vi "triggered scope simple.vi"() -> ()   [LabVIEW 2014]
uses:
  <vilib>/Utility/file.llb/Write To Spreadsheet File (DBL).vi
  <instrlib>/Tektronix TDS 200 1000 2000 Series/Public/Configure/Configure Trigger (Edge).vi
  <instrlib>/Tektronix TDS 200 1000 2000 Series/Public/Data/Read (Multiple Waveforms).vi
  <vilib>/Waveform/WDTOps.llb/WDT Waveform to XY Pairs DBL.vi
  <vilib>/Utility/file.llb/Write To Spreadsheet File (string).vi
  <instrlib>/Tektronix TDS 200 1000 2000 Series/Tektronix TDS 200 1000 2000 Series.lvlib
panel:
  in  "Pulse generator":T1={"Delay"={"A offset (s)"=0.0, "A reference"=enum."T0", "B reference"=enum."T0", "B offset (s)"=0.0, "C reference"=enum."T0", "C offset (s)"=0.0, "D reference"=enum."T0", "D offset (s)"=0.0}, "Trigger"={"Trigger"=enum."internal", "Burst count"=0, "Burst period"=0, "Input impedance"=FALSE, "Trigger slope"=FALSE, "Internal trigger rate"=0.001}, "Output"={"Mode"=enum."TTL", "Load"=FALSE, "Invert?"=FALSE, "Amplitude (V)"=2.0, "Offset (V)"=0.0, "Set output"=3}, "output cluster"={"mode"=0, "load"=FALSE, "inversion"=FALSE, "amplitude"=0.0, "offset"=0.0}} {"Output"."Set output" items=["T0", "A", "B", "AB", "C", "D", "CD"]; "Trigger"."Internal trigger rate" format="%#.9f"; "Trigger"."Burst period" max=1000 step=1; "Trigger"."Burst count" max=1000 step=1; "Delay"."D offset (s)" min=0.0 max=1.0; "Delay"."C offset (s)" min=0.0 max=1.0; "Delay"."B offset (s)" min=0.0 max=1.0; "Delay"."A offset (s)" min=0.0 max=1.0}
  out "File path":path
  in  "Tektronix scope":T2={"Trigger"={" Source"=4, "Level (V)"=0.5, "Trigger Mode"=1, "Trigger Coupling"=1, "Trigger on?"=TRUE}, "Channel 1"={"V/div"=2.0, " offset (V)"=0.0}, "Channel 2"={"V/div"=2.0, " offset (V)"=0.0}, "Time base"={"s/div"=0.003, " offset (s)"=0.0}} {"Time base"."offset (s)" min=-1.0 max=1.0; "Time base"."s/div" min=2.5e-09 max=50.0; "Channel 2"."offset (V)" min=-20.0 max=20.0; "Channel 2"."V/div" min=0.02 max=50.0; "Channel 1"."offset (V)" min=-20.0 max=20.0; "Channel 1"."V/div" min=0.02 max=50.0; "Trigger"."Trigger Coupling" items=["AC", "DC", "HF Reject", "LF Reject", "Noise Reject"]; "Trigger"."Trigger Mode" items=["Auto", "Normal"]; "Trigger"."Level (V)" min=0.0 max=4.0; "Trigger"."Source" items=["Channel 1", "Channel 2", "Channel 3", "Channel 4", "External Input", "Attenuated External Input"]}
  out "Waveform Graph":waveform(dbl)[](graph)
  in  "Stop Button":bool
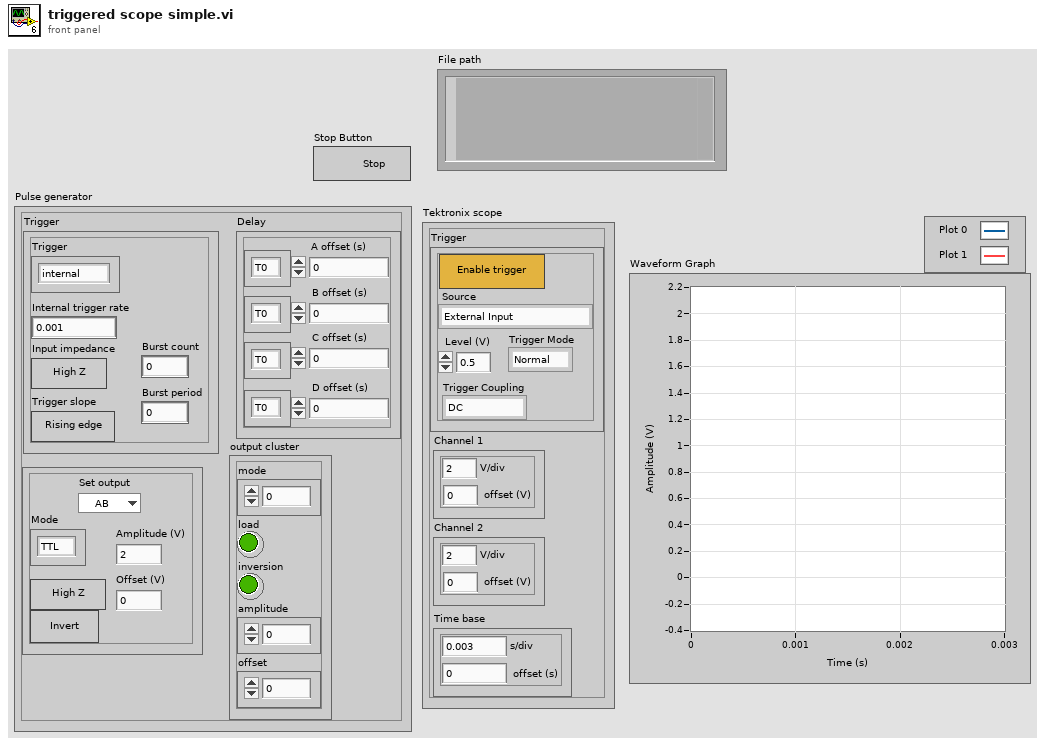
[diagram p1: front panel]
types:
  T1 = cluster{"Delay":cluster{"A offset (s)":dbl, "A reference":enum16{"T0", "B", "C", "D"}, "B reference":enum16{"T0", "A", "C", "D"}, "B offset (s)":dbl, "C reference":enum16{"T0", "A", "B", "D"}, "C offset (s)":dbl, "D reference":enum16{"T0", "A", "B", "C"}, "D offset (s)":dbl}, "Trigger":cluster{"Trigger":enum16{"internal", "external", "single shot", "burst", "line"}, "Burst count":u32, "Burst period":u32, "Input impedance":bool, "Trigger slope":bool, "Internal trigger rate":dbl}, "Output":cluster{"Mode":enum16{"TTL", "NIM", "ECL", "VAR"}, "Load":bool, "Invert?":bool, "Amplitude (V)":dbl, "Offset (V)":dbl, "Set output":u16}, "output cluster":cluster{"mode":u8, "load":bool, "inversion":bool, "amplitude":dbl, "offset":dbl}}
  T2 = cluster{"Trigger":cluster{" Source":i32, "Level (V)":dbl, "Trigger Mode":i32, "Trigger Coupling":i32, "Trigger on?":bool}, "Channel 1":cluster{"V/div":dbl, " offset (V)":dbl}, "Channel 2":cluster{"V/div":dbl, " offset (V)":dbl}, "Time base":cluster{"s/div":dbl, " offset (s)":dbl}}
  T3 = cluster{"Trigger":enum16{"internal", "external", "single shot", "burst", "line"}, "Burst count":u32, "Burst period":u32, "Input impedance":bool, "Trigger slope":bool, "Internal trigger rate":dbl}
  T4 = cluster{"A offset (s)":dbl, "A reference":enum16{"T0", "B", "C", "D"}, "B reference":enum16{"T0", "A", "C", "D"}, "B offset (s)":dbl, "C reference":enum16{"T0", "A", "B", "D"}, "C offset (s)":dbl, "D reference":enum16{"T0", "A", "B", "C"}, "D offset (s)":dbl}
  T5 = cluster{"Mode":enum16{"TTL", "NIM", "ECL", "VAR"}, "Load":bool, "Invert?":bool, "Amplitude (V)":dbl, "Offset (V)":dbl, "Set output":u16}
  T6 = enum16{"internal", "external", "single shot", "burst", "line"}
  T7 = cluster{" Source":i32, "Level (V)":dbl, "Trigger Mode":i32, "Trigger Coupling":i32, "Trigger on?":bool}
  T8 = cluster{"mode":u8, "load":bool, "inversion":bool, "amplitude":dbl, "offset":dbl}
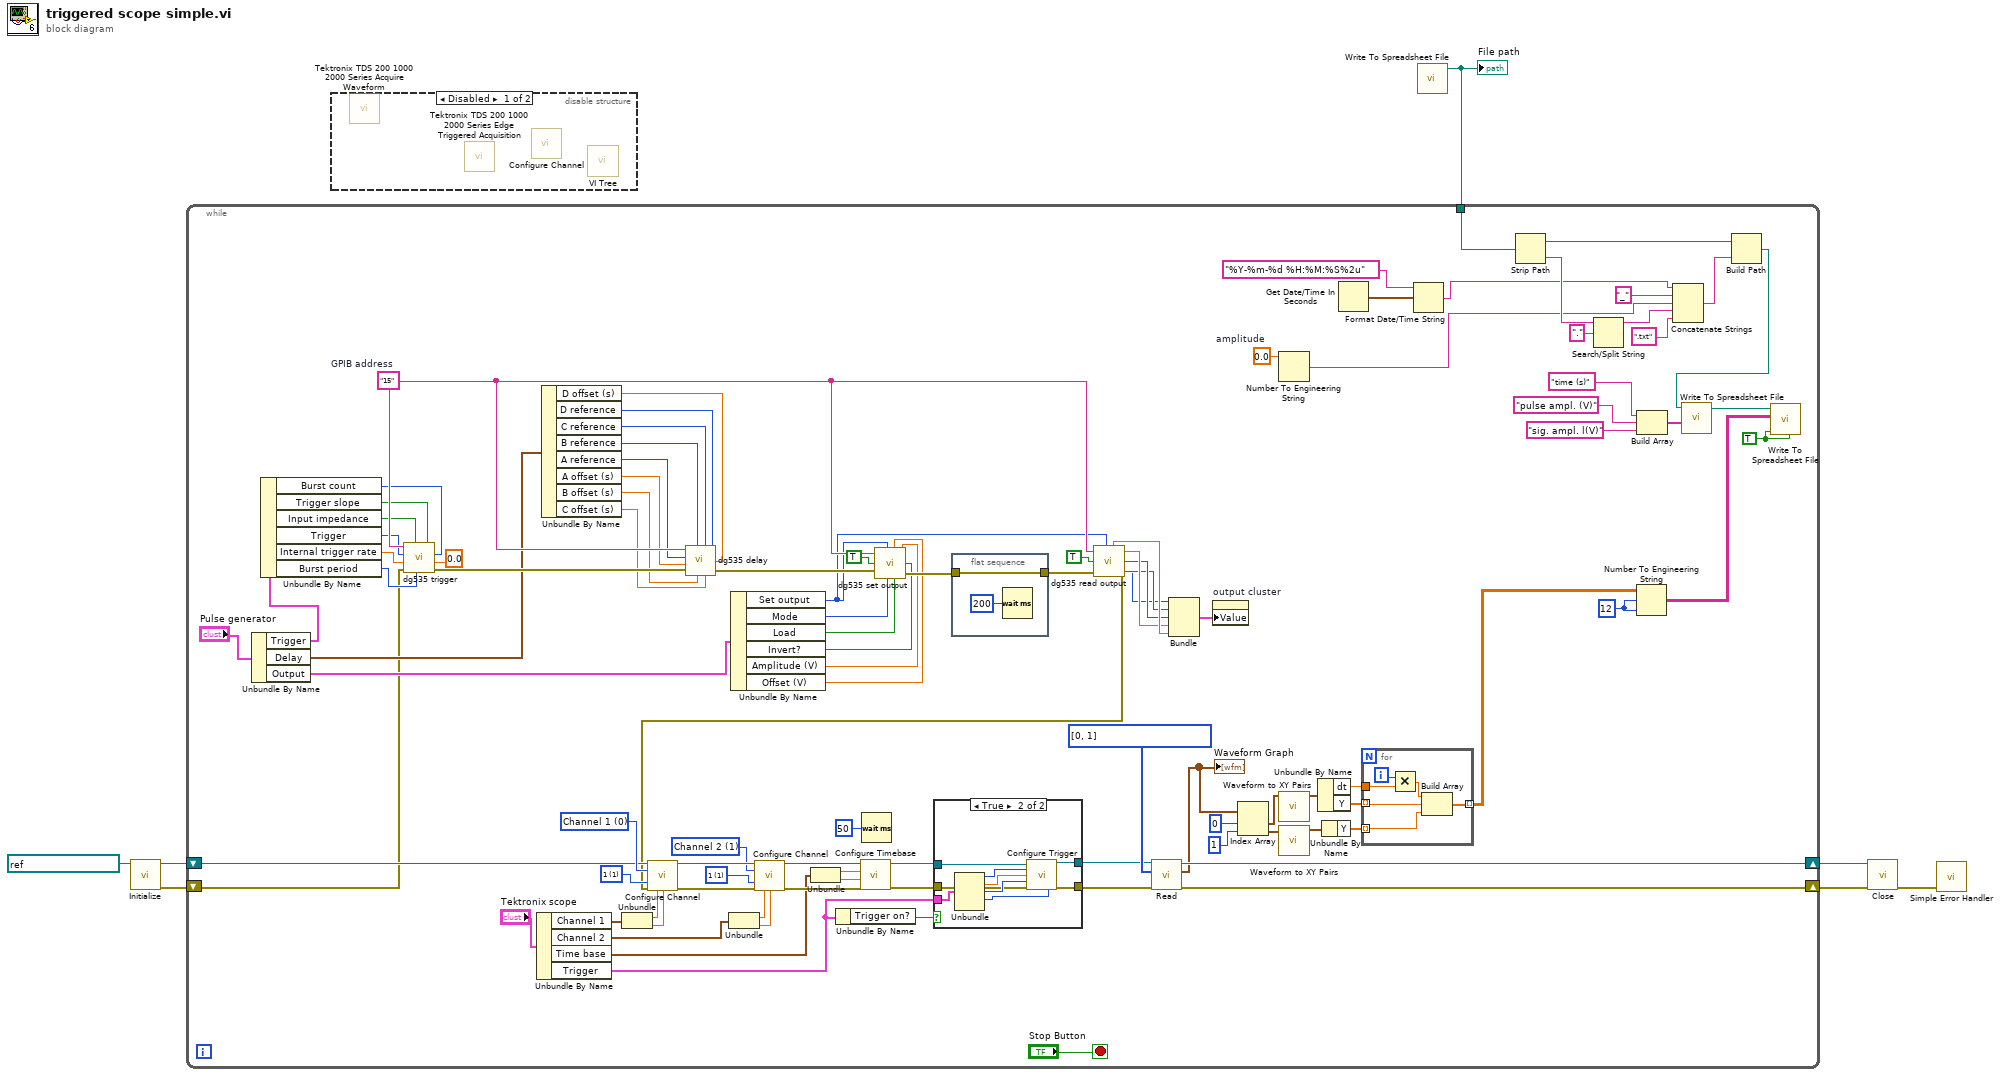
[diagram p0: block diagram]
diagram:
  n1 = call <instrlib>:"Initialize.vi"("VISA resource name"=refnum<visa-resource-name> "GPIB2::20::INSTR") -> ("error out"=w5:errorcluster, "VISA resource name out"=w6:refnum<visa-resource-name>)  [unwired: 9 in]
  n2 = disable-structure shown="Disabled" {
    frame Disabled {
      n3 = call "Tektronix TDS 200 1000 2000 Series Acquire Waveform.vi"() -> ()  [unwired: 1 in]
      n4 = call "Tektronix TDS 200 1000 2000 Series Edge Triggered Acquisition.vi"() -> ()  [unwired: 1 in]
      n5 = call <instrlib>:"Configure Channel.vi"() -> ()  [unwired: 14 in, 2 out]
      n6 = call "VI Tree.vi"() -> ()  [unwired: 12 in]
    }
    frame Enabled {
    }
  }
  n7 = call-poly <vilib>:"Write To Spreadsheet File.vi"() -> ("new file path (Not A Path if cancelled)"=w1:path)  [unwired: 8 in]
  "File path" <- w1
  n8 = while {
    shift-right: [w110] -> w7
    shift-left: w6 -> [w95]
    shift-right: [w109] -> w4
    shift-left: w5 -> [w9]
    tunnel: w1 -> [w57]
    stop <- "Stop Button" stop-if-true
    w36 = "15"  # GPIB address
    w48 = i16 12 ("width (-)")
    w52 = 0.0  # amplitude
    w58 = TRUE ("append to file? (new file:F)")
    w85 = 1 items=["1"=1, "10"=10, "20"=20, "50"=50, "100"=100, "500"=500, "1000"=1000] ("Probe Attenuation (10: 10X)")
    w87 = 1 items=["1"=1, "10"=10, "20"=20, "50"=50, "100"=100, "500"=500, "1000"=1000] ("Probe Attenuation (10: 10X)")
    w86 = u16 1 items=["Channel 1", "Channel 2", "Channel 3", "Channel 4", "Math", "Reference A", "Reference B", "Reference C", "Reference D", "FFT"] ("Source (0: Channel 1)")
    w100 = u16 0 items=["Channel 1", "Channel 2", "Channel 3", "Channel 4", "Math", "Reference A", "Reference B", "Reference C", "Reference D", "FFT"] ("Source (0: Channel 1)")
    w106 = u16[] [0, 1] items=["Channel 1", "Channel 2", "Channel 3", "Channel 4", "Math", "Reference A", "Reference B", "Reference C", "Reference D", "FFT"] ("Channels")
    n9 = Unbundle By Name("Pulse generator") -> ("Trigger"=w12:T3, "Delay"=w10:T4, "Output"=w11:T5)
    n10 = Unbundle By Name(w12) -> ("Burst count"=w26:u32, "Trigger slope"=w25:bool, "Input impedance"=w24:bool, "Trigger"=w23:T6, "Internal trigger rate"=w22:dbl, "Burst period"=w21:u32)
    n11 = call <instrlib>:"dg535 trigger.vi"("external trigger level"=sgl 0.0, "burst count"=w26, "trigger slope"=w25, "burst period"=w21, "input impedance"=w24, "error in"=w9, "internal/burst trigger rate"=w22, "trigger"=w23, "GPIB address"=w36) -> ("error out"=w47:errorcluster)
    n12 = Unbundle By Name("Tektronix scope") -> ("Channel 1"=w82:cluster{"V/div":dbl, " offset (V)":dbl}, "Channel 2"=w81:cluster{"V/div":dbl, " offset (V)":dbl}, "Time base"=w80:cluster{"s/div":dbl, " offset (s)":dbl}, "Trigger"=w79:T7)
    n13 = Unbundle By Name(w10) -> ("D offset (s)"=w35:dbl, "D reference"=w34:enum16{"T0", "A", "B", "C"}, "C reference"=w33:enum16{"T0", "A", "B", "D"}, "B reference"=w32:enum16{"T0", "A", "C", "D"}, "A reference"=w31:enum16{"T0", "B", "C", "D"}, "A offset (s)"=w30:dbl, "B offset (s)"=w29:dbl, "C offset (s)"=w28:dbl)
    n14 = Unbundle(w82) -> ("V/div"=w99:dbl, "offset (V)"=w98:dbl)
    n15 = call <instrlib>:"dg535 delay.vi"("C"=w28, "D"=w35, "D="=w34, "C="=w33, "B"=w29, "error in"=w47, "A"=w30, "B="=w32, "A="=w31, "GPIB address"=w36) -> ("error out"=w45:errorcluster)
    n16 = Unbundle(w81) -> ("V/div"=w97:dbl, "offset (V)"=w96:dbl)
    n17 = Unbundle By Name(w11) -> ("Set output"=w20:u16, "Mode"=w19:enum16{"TTL", "NIM", "ECL", "VAR"}, "Load"=w18:bool, "Invert?"=w17:bool, "Amplitude (V)"=w16:dbl, "Offset (V)"=w15:dbl)
    n18 = Unbundle(w80) -> ("s/div"=w92:dbl, "offset (s)"=w91:dbl)
    n19 = Unbundle By Name(w79) -> ("Trigger on?"=w88:bool)
    n20 = Wait (ms)(milliseconds to wait=u32 50) -> ()  [unwired: 1 out]
    n21 = call "dg535 set output.vi"("GPIB address"=w36, "output"=w20, "set"=TRUE, "error in"=w45, "mode"=w19, "offset"=w15, "amplitude"=w16, "inversion"=w17, "load"=w18) -> ("error out"=w38:errorcluster)
    n22 = flat-sequence {
      tunnel: w38 -> [w111]
      tunnel: [w111] -> w37
      frame #0 {
        n23 = Wait (ms)(milliseconds to wait=u32 200) -> ()  [unwired: 1 out]
      }
    }
    n24 = call "dg535 read output.vi"("GPIB address"=w36, "output"=w20, "read"=TRUE, "error in"=w37) -> ("mode"=w39:u8, "offset"=w43:dbl, "amplitude"=w42:dbl, "inversion"=w41:bool, "load"=w40:bool, "error out"=w8:errorcluster)
    n25 = call <instrlib>:"Configure Channel.vi"("VISA resource name"=w95, "Channel (0: Channel 1)"=w100, "Probe Attenuation (10: 10X)"=w87, "error in (no error)"=w8, "Vertical Range (10.0 V/div)"=w99, "Vertical Offset (0.0 divs)"=w98) -> ("VISA resource name out"=w105:refnum<visa-resource-name>, "error out"=w104:errorcluster)  [unwired: 8 in]
    n26 = call <instrlib>:"Configure Channel.vi"("VISA resource name"=w105, "Channel (0: Channel 1)"=w86, "Probe Attenuation (10: 10X)"=w85, "error in (no error)"=w104, "Vertical Range (10.0 V/div)"=w97, "Vertical Offset (0.0 divs)"=w96) -> ("VISA resource name out"=w94:refnum<visa-resource-name>, "error out"=w93:errorcluster)  [unwired: 8 in]
    n27 = call <instrlib>:"Configure Timebase.vi"("error in (no error)"=w93, "Position (0.0 s)"=w91, "Timebase (0.0005 s)"=w92, "VISA resource name"=w94) -> ("error out"=w89:errorcluster, "VISA resource name out"=w90:refnum<visa-resource-name>)  [unwired: 6 in]
    n28 = case shown="True" w88 {
      tunnel: w90 -> [w120 w125]
      tunnel: w89 -> [w119 w124]
      tunnel: [w120 w123] -> w73
      tunnel: [w119 w122] -> w72
      tunnel: w79 -> [_ w121]
      frame False {
      }
      frame True {
        n29 = Unbundle(w121) -> ("Source"=w126:i32, "Level (V)"=w127:dbl, "Trigger Mode"=w128:i32, "Trigger Coupling"=w129:i32)  [unwired: 1 out]
        n30 = call-poly <instrlib>:"Configure Trigger.vi"("VISA resource name"=w125, "Trigger Source (0: Channel 1)"=w126, "Trigger Level (0.0 V)"=w127, "Trigger Mode (0: Auto)"=w128, "error in (no error)"=w124, "Trigger Coupling (0: AC)"=w129) -> ("VISA resource name out"=w123:refnum<visa-resource-name>, "error out"=w122:errorcluster)  [unwired: 8 in]
      }
    }
    n31 = call-poly <instrlib>:"Read.vi"("error in (no error)"=w72, "Channels"=w106, "VISA resource name"=w73) -> ("error out"=w109:errorcluster, "Waveform Data"=w84:waveform(dbl)[], "VISA resource name out"=w110:refnum<visa-resource-name>)  [unwired: 6 in]
    "Waveform Graph" <- w84
    n32 = Bundle("mode"=w39, "load"=w40, "inversion"=w41, "amplitude"=w42, "offset"=w43) -> (w13:T8)  [unwired: 1 in]
    n33 = property on="output cluster" class="Clust (strict)"("Value"=w13) -> ()  [unwired: 2 in, 2 out]
    n34 = Index Array(array=w84, index #1=0 ("index"), index #2=1 ("index")) -> (element #1=w78:waveform(dbl), element #2=w101:waveform(dbl))
    n35 = Number To Engineering String(4:w52) -> (0:w53:string)  [unwired: 3 in]
    n36 = call-poly <vilib>:"Waveform to XY Pairs.vi"("waveform in"=w78) -> ("waveform out"=w77:waveform(dbl))  [unwired: 8 in, 2 out]
    n37 = call-poly <vilib>:"Waveform to XY Pairs.vi"("waveform in"=w101) -> ("waveform out"=w74:waveform(dbl))  [unwired: 8 in, 2 out]
    n38 = Unbundle By Name(w77) -> ("dt"=w76:dbl, "Y"=w75:dbl[])
    n39 = Unbundle By Name(w74) -> ("Y"=w70:dbl[])
    n40 = Get Date/Time In Seconds() -> (seconds since 1Jan1904=w71:timestamp)
    n41 = for {
      tunnel: w76 -> [w117]
      tunnel: w75 -> [w115] mode=indexing
      tunnel: [w114] -> w50 mode=indexing
      tunnel: w70 -> [w113] mode=indexing
      i -> [w118]
      n42 = Multiply(x=w118, y=w117) -> (x*y=w116:dbl)
      n43 = Build Array(w116, w115, w113) -> (w114:dbl[])
    }
    n44 = Format Date/Time String(time format string (%c)="%Y-%m-%d %H:%M:%S%2u", seconds (now)=w71) -> (date/time string=w55:string)  [unwired: 1 in]
    n45 = Strip Path(path=w57) -> (stripped path=w64:path, name=w63:string)
    n46 = Search/Split String(string=w63, search string/char (-)=".") -> (substring before match=w62:string)  [unwired: 1 in, 2 out]
    n47 = Number To Engineering String(2:w48, 3:w48, 4:w50) -> (0:w49:string[][])  [unwired: 1 in]
    n48 = Build Array("time (s)", "pulse ampl. (V)", "sig. ampl. l(V)") -> (w67:string[])
    n49 = Concatenate Strings(w55, "_" ("string"), w53, w62, ".txt" ("string")) -> (w60:string)
    n50 = Build Path(base path=w64, name or relative path=w60) -> (appended path=w68:path)
    n51 = call-poly <vilib>:"Write To Spreadsheet File.vi"("1D data"=w67, "file path (dialog if empty)"=w68) -> ("new file path (Not A Path if cancelled)"=w69:path)  [unwired: 6 in]
    n52 = call-poly <vilib>:"Write To Spreadsheet File.vi"("transpose? (no:F)"=w58, "append to file? (new file:F)"=w58, "2D data"=w49, "file path (dialog if empty)"=w69) -> ()  [unwired: 4 in, 1 out]
  }
  n53 = call <instrlib>:"Close.vi"("error in (no error)"=w4, "VISA resource name"=w7) -> ("error out"=w2:errorcluster)  [unwired: 9 in]
  n54 = call <vilib>:"Simple Error Handler.vi"("error in (no error)"=w2) -> ()  [unwired: 4 in, 5 out]
